vi "Write Goto.vi"(8 "error in (no error)":errorcluster, 9 "Enable warning? (T)":bool=TRUE, 10 "Target":dbl[unit], 11 "Power Supply in":refnum<class "Power Supply.lvclass">) -> (0 "error out":errorcluster, 3 "Power Supply out":refnum<class "Power Supply.lvclass">)   [LabVIEW 2023, in "Power Supply.lvclass"]
doc: "Tells magnet to now go to the target field (if Goto Zero is set to true, goes to 0 instead)."
uses:
  Power Supply.lvclass
  Power Supply.lvclass/Power Supply.ctl
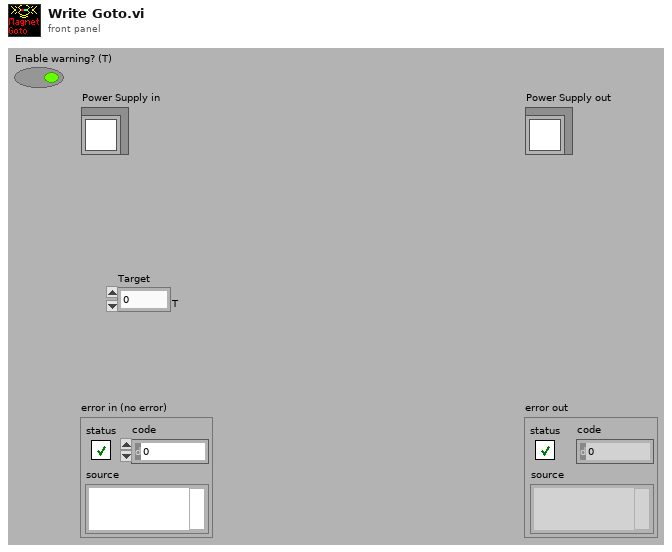
[diagram p1: front panel]
types:
  T1 = typedef "PSIO.ctl" = cluster{"Address":T2, "Version":enum16{"PS", "IPS"}}
  T2 = typedef "OxfordAddress.ctl" = cluster{"Com Port":i32, "ISOBUS Address":i32, "GPIB Address":i16, "Communication":enum16{"RS232", "ISOBUS", "GPIB", "Gateway"}}
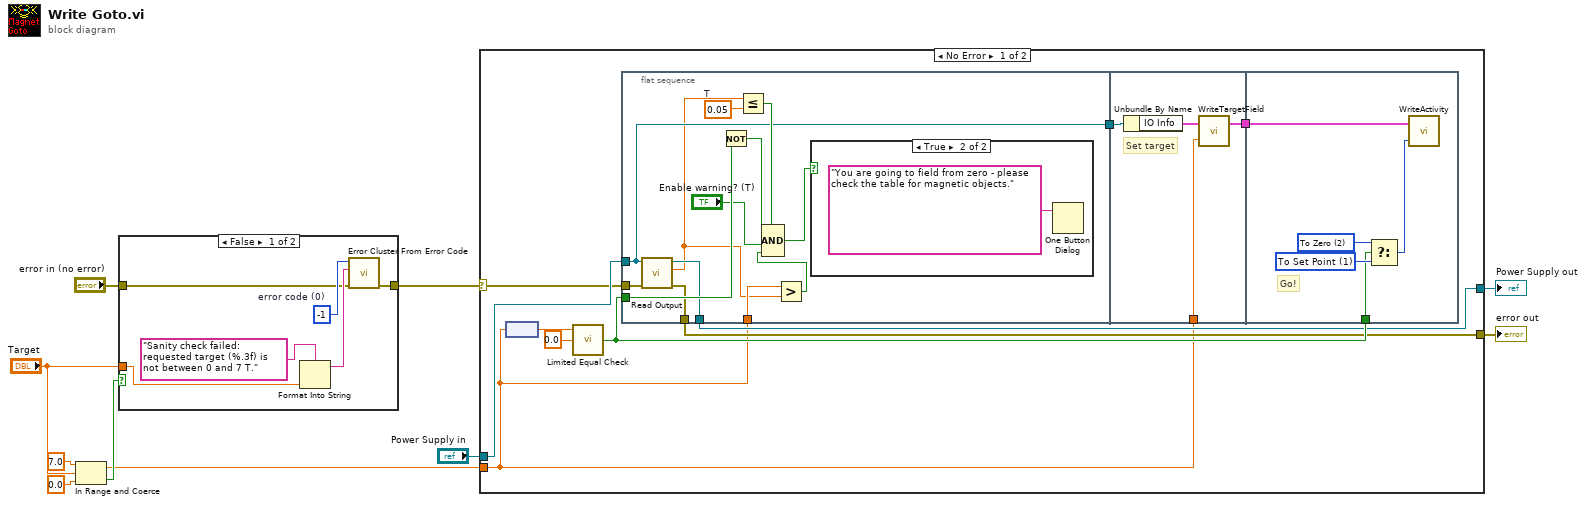
[diagram p0: block diagram]
diagram:
  n1 = In Range and Coerce(upper limit=dbl[unit] 7.0, x="Target", lower limit=dbl[unit] 0.0) -> (coerced(x)=w1:dbl[unit], In Range?=w3:bool)
  n2 = case shown="False" w3 {
    tunnel: [w16 w17] -> w5
    tunnel: "error in (no error)" -> [w11 w17]
    tunnel: "Target" -> [w13 _]
    frame False {
      w15 = -1  # error code (0)
      n3 = Format Into String(format string="Sanity check failed: requested target (%.3f) is not between 0 and 7 T." ("error message (\"\")"), w13) -> (resulting string=w12:string)  [unwired: 2 in, 1 out]
      n4 = call <vilib>:"Error Cluster From Error Code.vi"("error in (no error)"=w11, "error message (\"\")"=w12, "error code (0)"=w15) -> ("error out"=w16:errorcluster)  [unwired: 6 in]
    }
    frame True {
    }
  }
  n5 = case shown="No Error" w5 {
    selector: w5 -> [w20 w51]
    tunnel: "Power Supply in" -> [w23 w52]
    tunnel: [w22 w52] -> w9
    tunnel: [w21 w51] -> w8
    tunnel: w1 -> [w18 _]
    frame No Error {
      n6 = node(w18) -> (w19:dbl)
      n7 = call "Limited Equal Check.vi"("number2"=0.0, "number1"=w19) -> ("equal?"=w24:bool)  [unwired: 1 in, 2 out]
      n8 = flat-sequence {
        tunnel: [w34] -> w27
        tunnel: w24 -> [w36]
        tunnel: w23 -> [w34]
        tunnel: [w35] -> w22
        tunnel: w20 -> [w33]
        tunnel: [w32] -> w21
        tunnel: w18 -> [w29]
        tunnel: [w45] -> w26
        tunnel: w27 -> [w44]
        tunnel: w18 -> [w42]
        tunnel: w26 -> [w50]
        tunnel: w24 -> [w46]
        frame #0 {
          w40 = dbl[unit] 0.05  # T
          n9 = call-dynamic "Read Output.vi"("error in (no error)"=w33, "Power Supply in"=w34) -> ("error out"=w32:errorcluster, "Field"=w28:dbl[unit], "Power Supply out"=w35:refnum<class "Power Supply.lvclass">)  [unwired: 5 in, 2 out]
          n10 = Not(x=w36) -> (.not. x?=w37:bool)
          n11 = Less Or Equal?(x=w28, y=w40) -> (x <= y?=w39:bool)
          n12 = Greater?(x=w29, y=w28) -> (0:w30:bool)
          n13 = Compound Arithmetic op=AND(w39, w37, "Enable warning? (T)", w30) -> (w38:bool)
          n14 = case shown="True" w38 {
            frame False {
            }
            frame True {
              n15 = One Button Dialog(message="You are going to field from zero - please check the table for magnetic objects.") -> ()  [unwired: 2 out]
            }
          }
        }
        frame #1 {
          # "Set target"
          n16 = Unbundle By Name(w44) -> ("IO Info"=w43:T1)
          n17 = call "WriteTargetField.vi"("Target Field"=w42, "IO Info"=w43) -> ("IO Info"=w45:T1)  [unwired: 1 out]
        }
        frame #2 {
          w47 = u16 2 items=["Hold", "To Set Point", "To Zero", "Clamp"] ("Activity")
          w49 = u16 1 items=["Hold", "To Set Point", "To Zero", "Clamp"] ("Activity")
          # "Go!"
          n18 = Select(t=w47, s=w46, f=w49) -> (s? t:f=w48:u16)
          n19 = call "WriteActivity.vi"("Activity"=w48, "IO Info"=w50) -> ()  [unwired: 2 out]
        }
      }
    }
    frame Error {
    }
  }
  "error out" <- w8
  "Power Supply out" <- w9
